vi "Unflatten.vi"(8 "error in (no error)":errorcluster, 9 "timeout in":bool, 11 "CIFFifoCAN in":refnum<class "CIF_NIChn_FifoCAN.lvclass">) -> (0 "error out":errorcluster, 2 "Data":T1[](array[typedef]) {"Tags" format="%.0x"; "payload" format="%x"; "identifier" format="%x"}, 3 "CIFFifoCAN out":refnum<class "CIF_NIChn_FifoCAN.lvclass">, 4 "Header":T2)   [LabVIEW 2021, in "CIF_NIChn_FifoCAN.lvclass"]
uses:
  CIF_NIChn_FifoCAN.lvclass
  ChannelCommon/typedef/FIFO Header.ctl
  ChannelRegistrar/typedef/Datatype CAN.ctl
  CIF_NIChn_FifoCAN.lvclass/CIF_NIChn_FifoCAN.ctl
  ChannelCommon/CIFFIFO/CIFfifo.lvclass/CIFfifo.ctl
  ChannelCommon/CIFFIFO/Accessors/Read Header.vi
  ChannelCommon/CIFFIFO/Accessors/Write Header.vi
  ChannelCommon/CIFFIFO/CIFfifo.lvclass
  ChannelCommon/ChannelCommon.lvlib
  ChannelRegistrar/ChannelRegistrar.lvlib
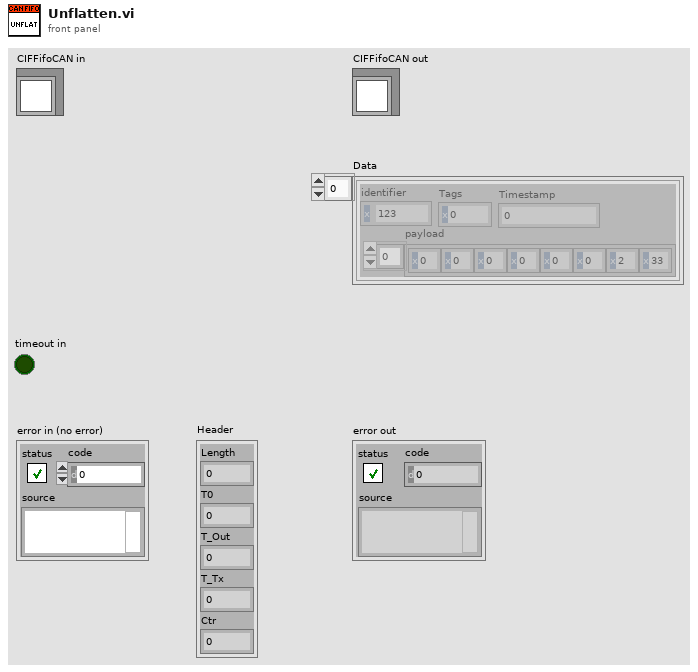
[diagram p1: front panel]
types:
  T1 = typedef "ChannelRegistrar.lvlib/Datatype CAN.ctl" = cluster{"payload":u8[], "identifier":u32, "Tags":u8, "Timestamp":u64}
  T2 = typedef "ChannelCommon.lvlib/FIFO Header.ctl" = cluster{"Length":u64, "T0":u64, "T_Out":u64, "T_Tx":u64, "Ctr":u64}
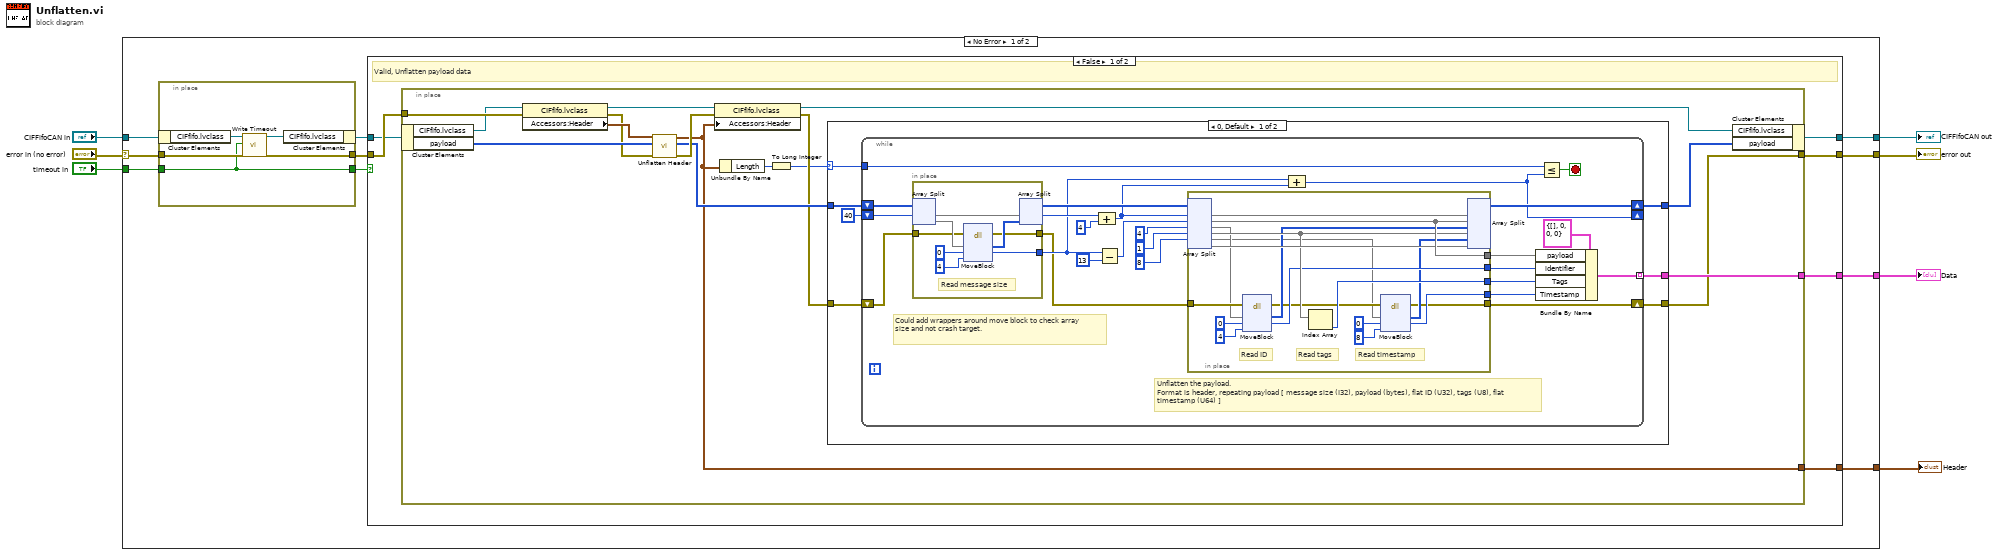
[diagram p0: block diagram]
diagram:
  n1 = case shown="No Error" "error in (no error)" {
    selector: "error in (no error)" -> [w16 w108]
    tunnel: [w9 w108] -> w6
    tunnel: [w10 w107] -> w4
    tunnel: "CIFFifoCAN in" -> [w17 w107]
    tunnel: "timeout in" -> [w15 _]
    tunnel: [w12 _] -> w1
    tunnel: [w11 _] -> w2
    frame No Error {
      n2 = in-place {
        in-place-border: w16 -> [w104]
        in-place-border: [w103] -> w14
        in-place-border: w15 -> [w102]
        in-place-border: [w102] -> w8
        n3 = in-place-cluster #1(w17) -> ("CIFfifo.lvclass"=w106:refnum<class "CIFfifo.lvclass">)
        n4 = call "Write Timeout.vi"("error in (no error)"=w104, "Timeout"=w102, "CIFFIFO in"=w106) -> ("error out"=w103:errorcluster, "CIFFIFO out"=w105:refnum<class "CIFfifo.lvclass">)  [unwired: 7 in]
        n5 = in-place-cluster #1("CIFfifo.lvclass"=w105) -> (w13:refnum<class "CIF_NIChn_FifoCAN.lvclass">)
      }
      n6 = case shown="False" w8 {
        tunnel: w14 -> [w23 w100]
        tunnel: w13 -> [w22 w101]
        tunnel: [w21 _] -> w12
        tunnel: [w20 _] -> w11
        tunnel: [w19 w101] -> w10
        tunnel: [w18 w100] -> w9
        frame False {
          # "Valid, Unflatten payload data"
          n7 = in-place {
            in-place-border: w23 -> [w38]
            in-place-border: [w26] -> w21
            in-place-border: [w30] -> w20
            in-place-border: [w25] -> w18
            n8 = in-place-cluster #2(w22) -> ("CIFfifo.lvclass"=w33:refnum<class "CIFfifo.lvclass">, "payload"=w39:u8[])
            n9 = property class="CIFfifo.lvclass"(reference=w33, error in=w38) -> (reference out=w35:refnum<class "CIFfifo.lvclass">, error out=w36:errorcluster, "Accessors:Header"=w37:T2)
            n10 = call "Unflatten Header.vi"("error in"=w36, "Flattened Data in"=w39, "Header in"=w37) -> ("error out"=w34:errorcluster, "Flatten Data out"=w31:u8[], "Header out"=w30:T2)  [unwired: 6 in]
            n11 = property class="CIFfifo.lvclass"(reference=w35, error in=w34, "Accessors:Header"=w30) -> (reference out=w32:refnum<class "CIFfifo.lvclass">, error out=w28:errorcluster)
            n12 = Unbundle By Name(w30) -> ("Length"=w29:u64)
            n13 = To Long Integer(number=w29) -> (32bit integer=w24:i32)
            n14 = case shown="0, Default" w24 {
              selector: w24 -> [w40 _]
              tunnel: w31 -> [w46 w99]
              tunnel: w28 -> [w45 w98]
              tunnel: [w44 w99] -> w27
              tunnel: [w43 _] -> w26
              tunnel: [w42 w98] -> w25
              frame 0, Default {
                n15 = while {
                  shift-right: [w54] -> w42
                  shift-left: w45 -> [w67]
                  shift-right: [w71] -> w44
                  shift-left: w46 -> [w69]
                  shift-right: [w50] -> _
                  shift-left: 40 -> [w68]
                  tunnel: [w52] -> w43 mode=indexing
                  tunnel: w40 -> [w51]
                  stop <- w49 stop-if-true
                  # "Could add wrappers around move block to check array size and not crash target."
                  # "Unflatten the payload.\nFormat is header, repeating payload [ message size (I32), payload (bytes), flat ID (U32), tags (U8), flat timestamp (U64) ]"
                  n16 = in-place {
                    in-place-border: w67 -> [w77]
                    in-place-border: [w73] -> w60
                    in-place-border: [w72] -> w48
                    # "Read message size"
                    n17 = in-place-split #3(w69, w68) -> (w79:u8[], w78:u8[])
                    n18 = dll-call lib="LabVIEW" fn="MoveBlock"(error in=w77, "source"=w78, "dest"=0, "size"=u64 4) -> (error out=w72:errorcluster, "source"=w74:u8[], "dest"=w73:i32)  [unwired: 4 in, 1 out]
                    n19 = in-place-split #3(w79, w74) -> (w65:u8[], w66:i32)
                  }
                  n20 = Compound Arithmetic op=ADD(w66, 4 ("value")) -> (w61:i32)
                  n21 = Subtract(x=w60, y=13) -> (x-y=w62:i32)
                  n22 = in-place {
                    in-place-border: [w96] -> w58
                    in-place-border: [w87] -> w56
                    in-place-border: [w94] -> w55
                    in-place-border: [w80] -> w54
                    in-place-border: w48 -> [w92]
                    in-place-border: [w81] -> w53
                    # "Read timestamp"
                    # "Read tags"
                    # "Read ID"
                    n23 = in-place-split #4(w65, w61, w62, 4, 1, 8) -> (w97:u8[], w96:u8[], w91:u8[], w93:u8[], w83:u8[], w95:u8[])
                    n24 = dll-call lib="LabVIEW" fn="MoveBlock"(error in=w92, "source"=w91, "dest"=u32 0, "size"=u64 4) -> (error out=w85:errorcluster, "source"=w88:u8[], "dest"=w87:u32)  [unwired: 4 in, 1 out]
                    n25 = Index Array(array=w93) -> (element=w94:u8)  [unwired: 1 in]
                    n26 = dll-call lib="LabVIEW" fn="MoveBlock"(error in=w85, "source"=w83, "dest"=u64 0, "size"=u64 8) -> (error out=w80:errorcluster, "source"=w82:u8[], "dest"=w81:u64)  [unwired: 4 in, 1 out]
                    n27 = in-place-split #4(w97, w96, w88, w93, w82, w95) -> (w71:u8[])  [unwired: 5 out]
                  }
                  n28 = Compound Arithmetic op=ADD(w60, w61) -> (w50:i32)
                  n29 = Bundle By Name(cluster=T1 {"payload"=[], "identifier"=0, "Tags"=0, "Timestamp"=0} ("Data"), "payload"=w58, "identifier"=w56, "Tags"=w55, "Timestamp"=w53) -> (w52:T1)
                  n30 = Less Or Equal?(x=w51, y=w50) -> (x <= y?=w49:bool)
                }
              }
              frame 40 {
                # "Empty message (only header)"
              }
            }
            n31 = in-place-cluster #2("CIFfifo.lvclass"=w32, "payload"=w27) -> (w19:refnum<class "CIF_NIChn_FifoCAN.lvclass">)
          }
        }
        frame True {
          # "Timeout"
        }
      }
    }
    frame Error {
    }
  }
  "error out" <- w6
  "CIFFifoCAN out" <- w4
  "Header" <- w2
  "Data" <- w1
